vi "TDMS Logger.vi"() -> ()   [LabVIEW 2010]
panel:
  out "Time Data":waveform(dbl)[](graph)
  out "Power Spectrum":waveform(dbl)[](graph)
  in  "UUT Serial Numbers":string[](array[string])
  in  "Test Operator":string
  in  "TDMS File Path":path=path "D:/NI eLearning/LV Core 2/Using TDMS Files/Exercise/Test Data.tdms"
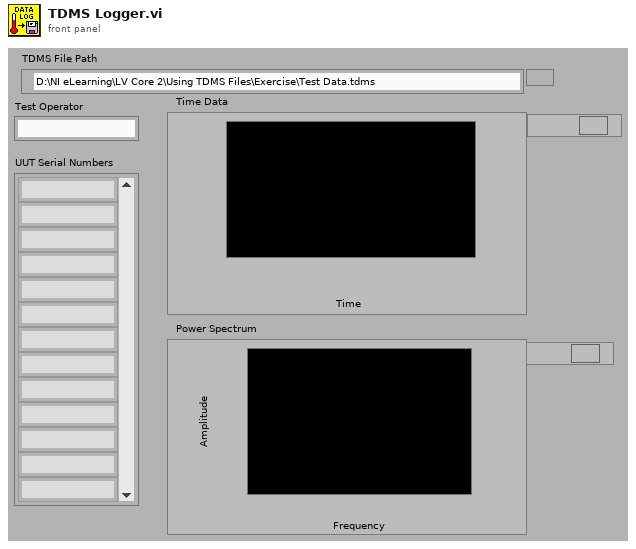
[diagram p1: front panel]
types:
  T1 = enum16{"open", "open or create", "create or replace", "create", "open (read-only)"}
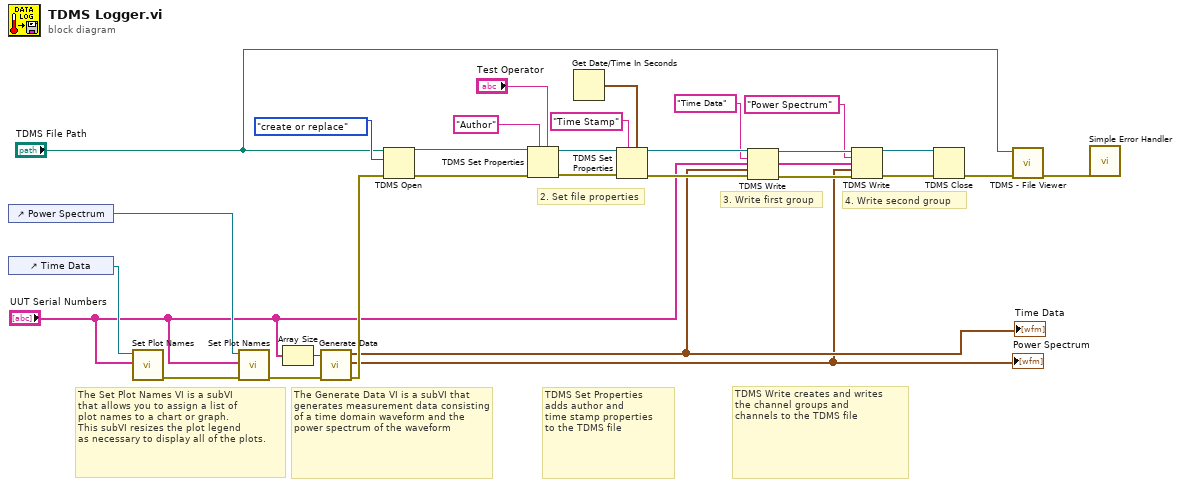
[diagram p0: block diagram]
diagram:
  # "4. Write second group"
  # "3. Write first group"
  # "2. Set file properties"
  # "TDMS Set Properties \nadds author and \ntime stamp properties \nto the TDMS file"
  # "TDMS Write creates and writes \nthe channel groups and\nchannels to the TDMS file"
  # "The Generate Data VI is a subVI that\ngenerates measurement data consisting\nof a time domain waveform and the \npower spectrum of the waveform"
  # "The Set Plot Names VI is a subVI\nthat allows you to assign a list of\nplot names to a chart or graph.\nThis subVI resizes the plot legend\nas necessary to display all of the plots."
  n1 = control-ref of="Power Spectrum"() -> (w30:refnum<vi>)
  n2 = control-ref of="Time Data"() -> (w26:refnum<vi>)
  n3 = call "Set Plot Names.vi"("Plot Names"="UUT Serial Numbers", "Graph Reference"=w26) -> ("error out"=w29:errorcluster)  [unwired: 9 in]
  n4 = call "Set Plot Names.vi"("error in (no error)"=w29, "Plot Names"="UUT Serial Numbers", "Graph Reference"=w30) -> ("error out"=w27:errorcluster)  [unwired: 8 in]
  n5 = Array Size(array="UUT Serial Numbers") -> (size(s)=w28:i32)
  n6 = call "Generate Data.vi"("error in"=w27, "Number of Channels"=w28) -> ("error out"=w24:errorcluster, "Power Spectrum Data"=w9:waveform(dbl)[], "Waveform Chart"=w13:waveform(dbl)[])  [unwired: 7 in]
  "Power Spectrum" <- w9
  "Time Data" <- w13
  n7 = TDMS Open(8:w24, 10:T1."create or replace" ("operation (0:open)"), 11:"TDMS File Path") -> (0:w18:errorcluster, 3:w23:refnum<k34>)  [unwired: 3 in]
  n8 = TDMS Set Properties(5:"Test Operator", 7:"Author", 8:w18, 11:w23) -> (0:w22:errorcluster, 3:w21:refnum<k34>)  [unwired: 2 in, 2 out]
  n9 = Get Date/Time In Seconds() -> (seconds since 1Jan1904=w19:timestamp)
  n10 = TDMS Set Properties(5:w19, 7:"Time Stamp" ("Title"), 8:w22, 11:w21) -> (0:w16:errorcluster, 3:w17:refnum<k34>)  [unwired: 2 in, 2 out]
  n11 = TDMS Write(0:w17, 5:"Time Data" ("group name in (Untitled)"), 7:"UUT Serial Numbers", 9:w13, 11:w16) -> (4:w12:refnum<k34>, 8:w8:string[], 15:w11:errorcluster)  [unwired: 1 in, 1 out]
  n12 = TDMS Write(0:w12, 5:"Power Spectrum" ("group name in (Untitled)"), 7:w8, 9:w9, 11:w11) -> (4:w7:refnum<k34>, 15:w6:errorcluster)  [unwired: 1 in, 2 out]
  n13 = TDMS Close(8:w6, 11:w7) -> (0:w5:errorcluster)  [unwired: 1 out]
  n14 = call <vilib>:"TDMS - File Viewer.vi"("error in (no error)"=w5, "file path"="TDMS File Path") -> ("error out"=w3:errorcluster)  [unwired: 4 in, 1 out]
  n15 = call <vilib>:"Simple Error Handler.vi"("error in (no error)"=w3) -> ()  [unwired: 4 in, 5 out]
